vi "ATSh_GetBoardKind.vi"(11 "HandleIn":u32) -> (2 "ID":i32, 3 "HandleOut":u32)   [LabVIEW 2010]
doc: "_____AlazarTech, Scope_____\n\nRetrieve the board type identifier.\n\nInput:\n\"HandleIn\" = device to retrieve information\n\nOutput:\n\"HandleOut\" = device information\n\"Version\" = version\n\"ID\" = board identifications"
uses:
  ATSApi.dll
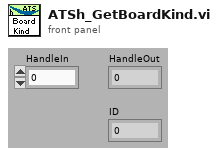
[diagram p1: front panel]
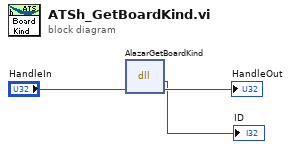
[diagram p0: block diagram]
diagram:
  n1 = dll-call lib="ATSApi.dll" fn="AlazarGetBoardKind"("h"="HandleIn") -> (→"ID":u32, "h"=→"HandleOut":u32)  [unwired: 3 in, 2 out]
